vi "Write Name Library File Path.vi"(10 "Name Library File Path":path, 11 "_Rescript Msg in":refnum<class "_Msg Rescript.lvclass">) -> (3 "_Rescript Msg out":refnum<class "_Msg Rescript.lvclass">)   [LabVIEW 2025, in "_Msg Rescript.lvlib" / "_Msg Rescript.lvclass"]
uses:
  _Msg Rescript.lvclass
  _Msg Rescript.lvclass/_Msg Rescript.ctl
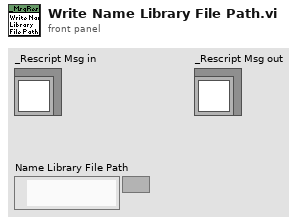
[diagram p1: front panel]
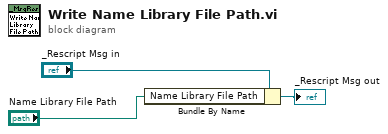
[diagram p0: block diagram]
diagram:
  n1 = Bundle By Name(cluster="_Rescript Msg in", "Name Library File Path"="Name Library File Path") -> (→"_Rescript Msg out":refnum<class "_Msg Rescript.lvclass">)
